vi "Insert Into Subpanel.vi"(8 "Error In":errorcluster, 10 "SubPanel Ref":refnum<vi>, 11 "Subpanel Inserter":refnum<class "Subpanel Inserter.lvclass">) -> (0 "error out":errorcluster, 3 "Subpanel Inserter":refnum<class "Subpanel Inserter.lvclass">)   [LabVIEW 2014, in "Subpanel Insertion.lvlib" / "Subpanel Inserter.lvclass"]
uses:
  Subpanel Inserter.lvclass
panel:
  out "NaN/Path/Refnum?":bool
  out "Already vi in subpanel":bool
  out "class name":string
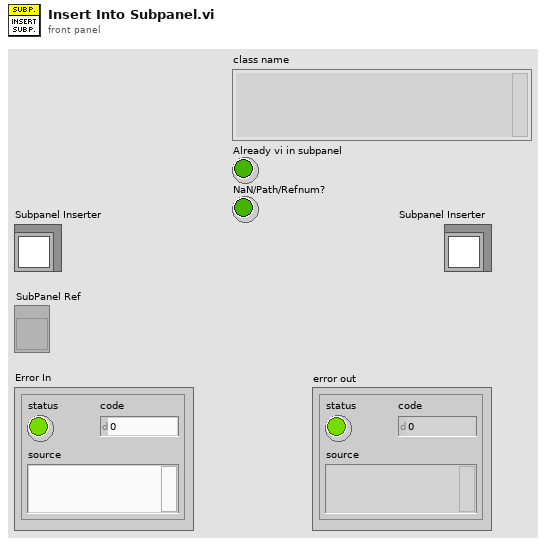
[diagram p1: front panel]
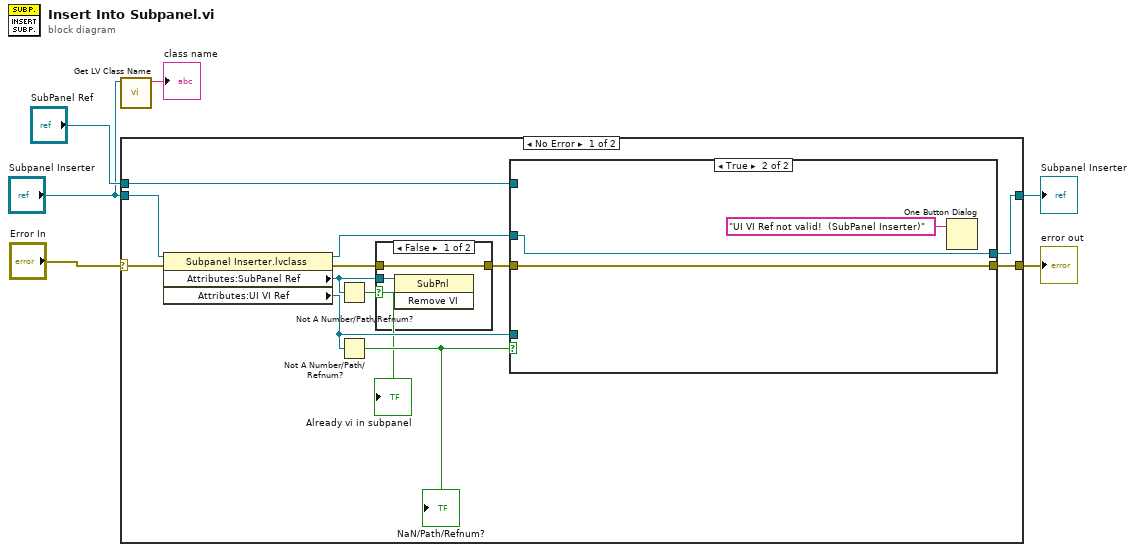
[diagram p0: block diagram]
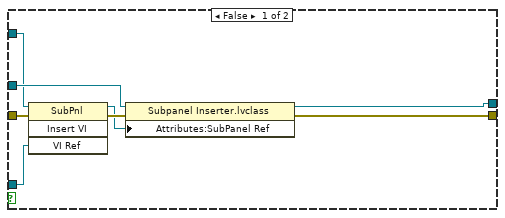
[diagram p2: hidden frame]
diagram:
  n1 = call <vilib>:"Get LV Class Name.vi"("object"="Subpanel Inserter") -> ("class name"=→"class name":string)  [unwired: 9 in, 1 out]
  n2 = case shown="No Error" "Error In" {
    selector: "Error In" -> [w17 w33]
    tunnel: "Subpanel Inserter" -> [w18 w34]
    tunnel: "SubPanel Ref" -> [w13 _]
    tunnel: [w12 w34] -> w3
    tunnel: [w11 w33] -> w4
    frame No Error {
      n3 = property class="Subpanel Inserter.lvclass"(reference=w18, error in=w17) -> (reference out=w16:refnum<class "Subpanel Inserter.lvclass">, error out=w8:errorcluster, "Attributes:SubPanel Ref"=w10:refnum<vi>, "Attributes:UI VI Ref"=w14:refnum<vi>)
      n4 = Not A Number/Path/Refnum?(number/path/refnum=w10) -> (NaN/Path/Refnum?=w9:bool)
      "Already vi in subpanel" <- w9
      n5 = Not A Number/Path/Refnum?(number/path/refnum=w14) -> (NaN/Path/Refnum?=w15:bool)
      "NaN/Path/Refnum?" <- w15
      n6 = case shown="False" w9 {
        tunnel: w10 -> [w31 _]
        tunnel: w8 -> [w30 w32]
        tunnel: [w30 w32] -> w7
        frame False {
          n7 = invoke on="Invoke Node" class="SubPnl" method="Remove VI"(reference=w31) -> ()  [unwired: 2 in, 3 out]
        }
        frame True {
        }
      }
      n8 = case shown="True" w15 {
        tunnel: w16 -> [w26 w29]
        tunnel: w14 -> [w19 _]
        tunnel: w13 -> [w23 _]
        tunnel: w7 -> [w22 w28]
        tunnel: [w25 w29] -> w12
        tunnel: [w24 w28] -> w11
        frame False {
          n9 = invoke class="SubPnl" method="Insert VI"(reference=w23, error in=w22, "VI Ref"=w19) -> (reference out=w20:refnum<vi>, error out=w21:errorcluster)  [unwired: 1 in, 2 out]
          n10 = property class="Subpanel Inserter.lvclass"(reference=w26, error in=w21, "Attributes:SubPanel Ref"=w20) -> (reference out=w25:refnum<class "Subpanel Inserter.lvclass">, error out=w24:errorcluster)
        }
        frame True {
          n11 = One Button Dialog(message="UI VI Ref not valid!  (SubPanel Inserter)") -> ()  [unwired: 1 in, 1 out]
        }
      }
    }
    frame Error {
    }
  }
  "error out" <- w4
  "Subpanel Inserter" <- w3
